vi "Test_010620.vi"() -> ()   [LabVIEW 2020]
panel:
  out "?":dbl
  out "Farenheight":dbl
  out "Temperature Graph":dbl[](graph)
  in  "?":bool
  out "Temperature Chart":dbl(graph)
  in  "Convert to celcius":bool
  in  "Thermometer F":dbl(slide) scale=0.0..100.0
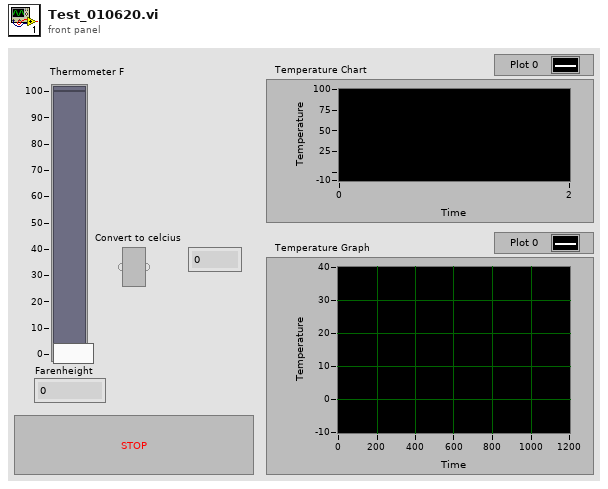
[diagram p1: front panel]
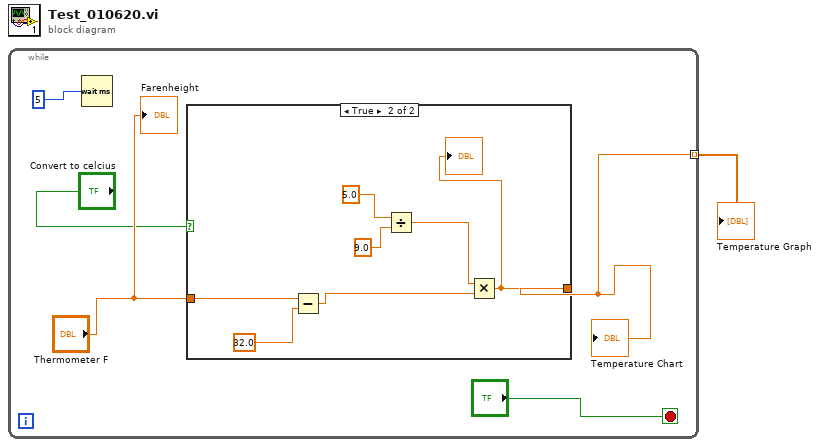
[diagram p0: block diagram]
diagram:
  n1 = while {
    tunnel: [w2] -> w1 mode=indexing
    stop <- "?" stop-if-true
    n2 = Wait (ms)(milliseconds to wait=u32 5) -> ()  [unwired: 1 out]
    n3 = case shown="True" "Convert to celcius" {
      tunnel: [w7 w8] -> w2
      tunnel: "Thermometer F" -> [w7 w9]
      frame False {
      }
      frame True {
        n4 = Subtract(x=w9, y=32.0) -> (x-y=w10:dbl)
        n5 = Divide(x=5.0, y=9.0) -> (x/y=w11:dbl)
        n6 = Multiply(x=w11, y=w10) -> (x*y=w8:dbl)
        "?" <- w8
      }
    }
    "Temperature Chart" <- w2
    "Farenheight" <- "Thermometer F"
  }
  "Temperature Graph" <- w1
